vi "m10.wfg.01DC.vi"(1 "Param 0":dbl=1000.0, 2 "Param 1":dbl, 3 "Param 2":dbl, 4 "Param 3":dbl, 5 "error in (no error)":errorcluster, 8 "Waveform Properties":T1={"Fs (Hz)"=20000.0, "Amplitude (V)"=5.0, "Ramp (s)"=0.02} {"Ramp (s)" min=0.0; "Fs (Hz)" min=0.0}, 10 "Duration (s)":dbl=0.1) -> (14 "Waveform Out":waveform(dbl), 19 "error out":errorcluster)   [LabVIEW 2013]
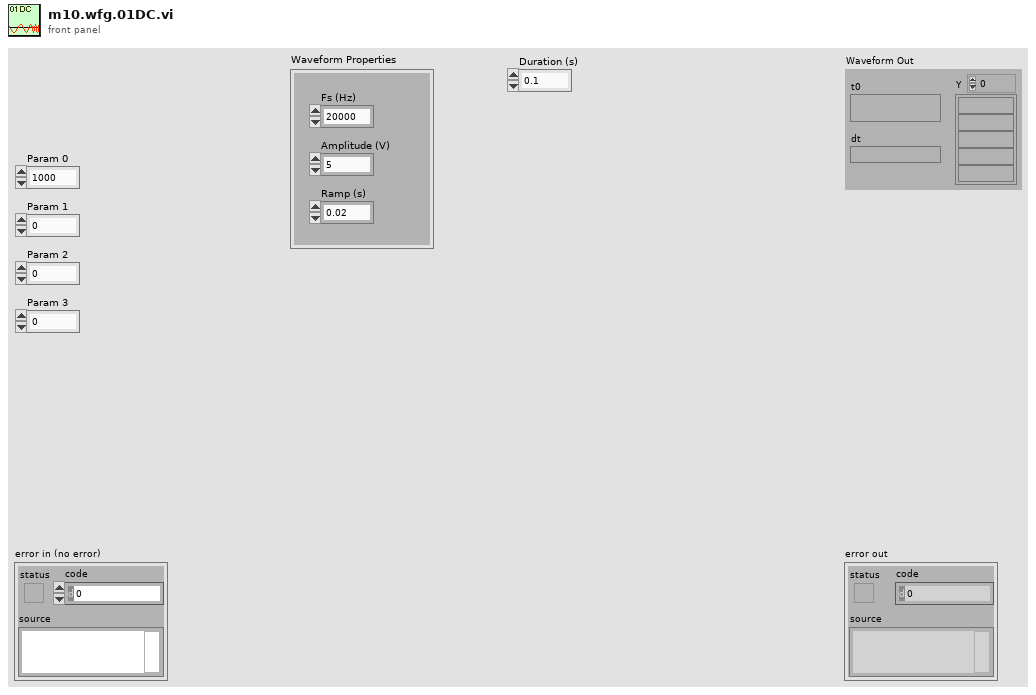
[diagram p1: front panel]
types:
  T1 = cluster{"Fs (Hz)":dbl, "Amplitude (V)":dbl, "Ramp (s)":dbl}
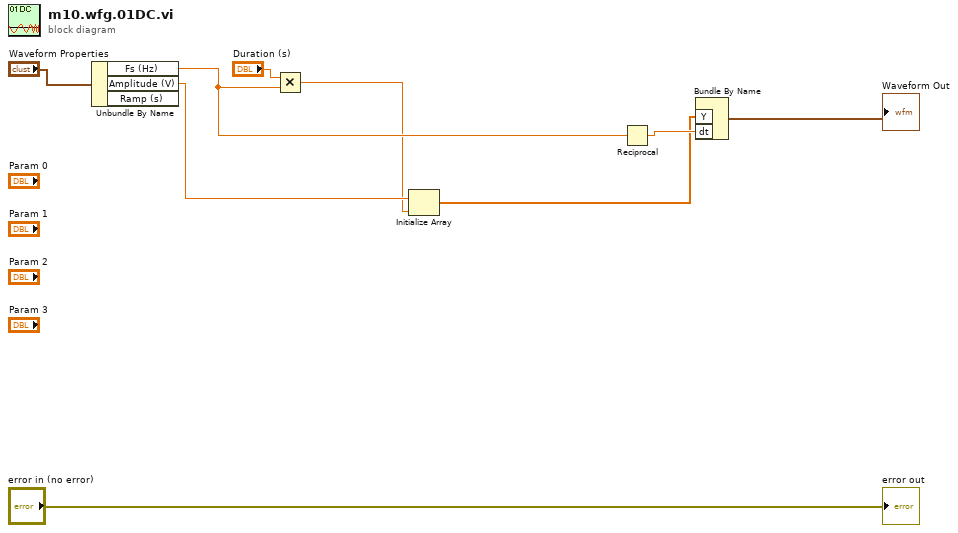
[diagram p0: block diagram]
diagram:
  n1 = Unbundle By Name("Waveform Properties") -> ("Fs (Hz)"=w5:dbl, "Amplitude (V)"=w4:dbl)  [unwired: 1 out]
  n2 = Multiply(x="Duration (s)", y=w5) -> (x*y=w3:dbl)
  n3 = Initialize Array(w4, w3) -> (w2:dbl[])
  n4 = Reciprocal(x=w5) -> (1/x=w8:dbl)
  n5 = Bundle By Name("Y"=w2, "dt"=w8) -> (→"Waveform Out":waveform(dbl))  [unwired: 1 in]
  "error out" <- "error in (no error)"
